vi "event structure 13.vi"() -> ()   [LabVIEW 2025]
panel:
  in  "stop":bool
  in  "b":dbl(slide) scale=0.0..10.0
  in  "a":dbl(slide) scale=0.0..10.0
  out "Tank":dbl(slide) scale=0.0..10.0
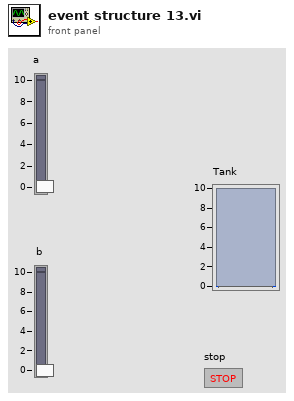
[diagram p1: front panel]
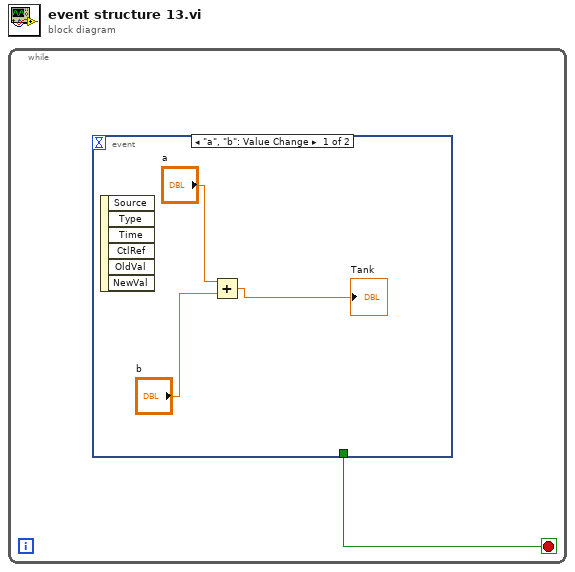
[diagram p0: block diagram]
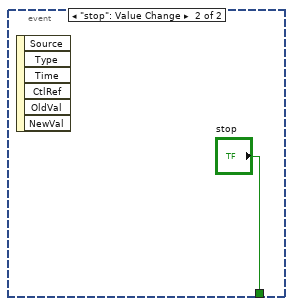
[diagram p2: hidden frame]
diagram:
  n1 = while {
    stop <- w1 stop-if-true
    n2 = event shown="[0] \"a\", \"b\": Value Change" {
      selector: _ -> [_ _]
      dyn-events: _ -> [_ _]
      timeout: _ -> [_ _]
      tunnel: [_ "stop"] -> w1
      event "a", "b": Value Change {
        n3 = event-data() -> ()  [unwired: 1 in, 6 out]
        n4 = Add(x="a", y="b") -> (x+y=→"Tank":dbl)
      }
      event "stop": Value Change {
        n5 = event-data() -> ()  [unwired: 1 in, 6 out]
      }
    }
  }
